vi "Populate Scope.vi"(8 "Error In":errorcluster, 11 "State In":T1) -> (0 "Error Out":errorcluster, 3 "State Out":T1)   [LabVIEW 2017, in "Graveyard.lvlib"]
uses:
  Graveyard.lvlib
  State.ctl
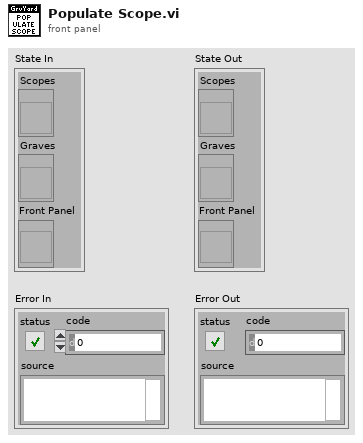
[diagram p1: front panel]
types:
  T1 = typedef "Graveyard.lvlib/State.ctl" = cluster{"Scopes":refnum<vi>, "Graves":refnum<vi>, "Front Panel":refnum<vi>}
  T2 = enum8{"Enabled", "Disabled", "Disabled and Grayed Out"}
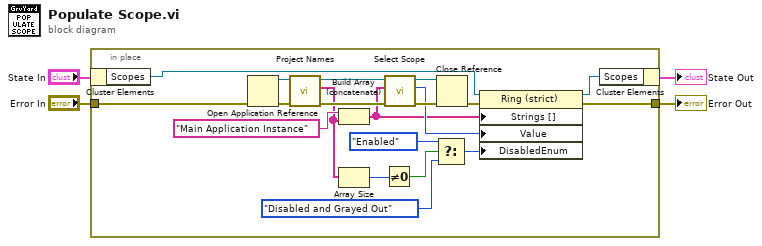
[diagram p0: block diagram]
diagram:
  n1 = in-place {
    in-place-border: "Error In" -> [w22]
    in-place-border: [w23] -> w3
    n2 = in-place-cluster #1("State In") -> ("Scopes"=w7:refnum<vi>)
    n3 = Open Application Reference(8:w22) -> (0:w21:errorcluster, 3:w20:refnum<vi>)  [unwired: 3 in]
    n4 = call "Project Names.vi"("Error In"=w21, "App In"=w20) -> ("Error Out"=w18:errorcluster, "Project Names"=w10:string[], "App Out"=w19:refnum<vi>)  [unwired: 7 in]
    n5 = Build Array (concatenate)("Main Application Instance", w10) -> (w5:string[])
    n6 = Array Size(array=w10) -> (size(s)=w9:i32)
    n7 = Not Equal To 0?(x=w9) -> (x != 0?=w8:bool)
    n8 = call "Select Scope.vi"("Error In"=w18, "Strings[]"=w5, "App In"=w19) -> ("Error Out"=w15:errorcluster, "Selection"=w6:u16, "App Out"=w16:refnum<vi>)  [unwired: 6 in]
    n9 = Select(t=T2."Enabled" ("Disabled"), s=w8, f=T2."Disabled and Grayed Out" ("Disabled")) -> (s? t:f=w12:T2)
    n10 = Close Reference(reference=w16, error in (no error)=w15) -> (error out=w17:errorcluster)
    n11 = property class="Ring (strict)"(reference=w7, error in=w17, "Strings []"=w5, "Value"=w6, "DisabledEnum"=w12) -> (reference out=w24:refnum<vi>, error out=w23:errorcluster)
    n12 = in-place-cluster #1("Scopes"=w24) -> (→"State Out":T1)
  }
  "Error Out" <- w3
